vi "Simple Server.vi"() -> ()   [LabVIEW 2020]
uses:
  source/PV Data/NT Scalar (Numeric)/NT Scalar (Numeric).lvclass
  C:/Users/eyw68381/source/repos/pvaccess-labview/labview/source/PV Data/NT Scalar/NT Scalar.lvclass
  C:/Users/eyw68381/source/repos/pvaccess-labview/labview/source/PV Data/NT Base/NT Base.lvclass
  source/PV Data/NT Scalar/NT Scalar.lvclass
  source/PV Data/PV Data/PV Data.lvclass
  source/Server/Server/Server.lvclass
  source/Server/Source/Source.lvclass
  7054ff5f-c778-4b9f-bf9e-4a55a1cdcc59.vi
  4fabb87d-4e15-4188-883f-208453235fd8.vi
  6c06fff3-e822-4e92-b24f-bdc271668697.vi
  0073a8bc-0586-4490-b945-e374f2b6411c.vi
  50f37ae9-e558-497d-927d-4042e789ec73.vi
panel:
  in  "PV name":string="DEV:SIMPLE_TEST"
  out "timestamp":timestamp
  in  "Value":dbl min=0.0 max=10.0 step=0.5 format="%.3f"
  in  "Increment":bool
  in  "stop":bool
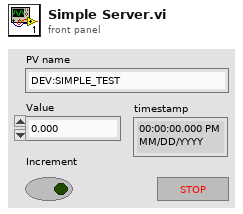
[diagram p1: front panel]
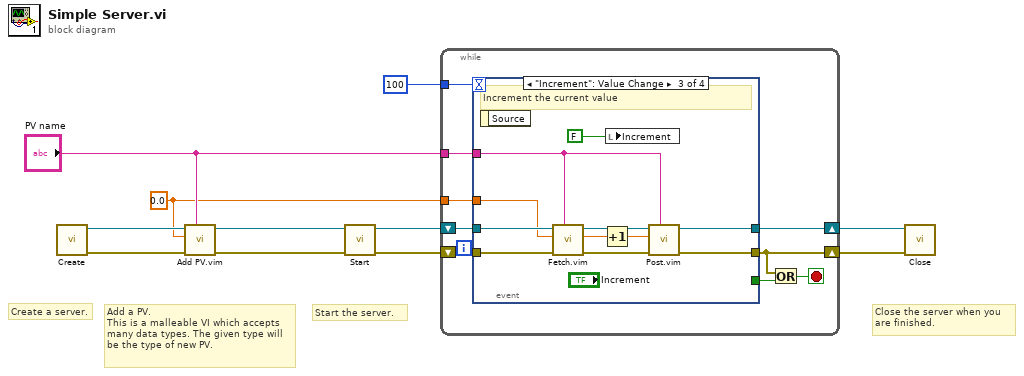
[diagram p0: block diagram]
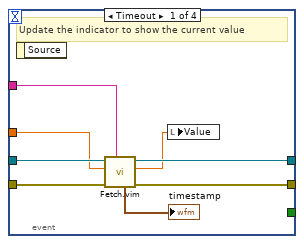
[diagram p2: hidden frame]
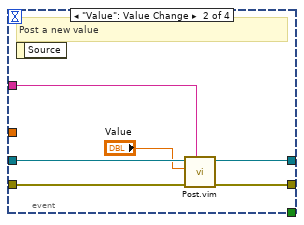
[diagram p3: hidden frame]
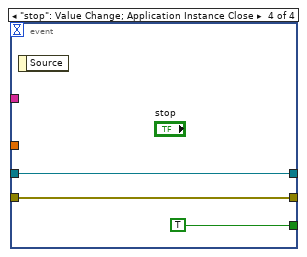
[diagram p4: hidden frame]
diagram:
  w1 = 0.0
  # "Close the server when you are finished."
  # "Start the server."
  # "Add a PV.\nThis is a malleable VI which accepts many data types. The given type will be the type of new PV."
  # "Create a server."
  n1 = call "Create.vi"() -> ("error out"=w2:errorcluster, "Server out"=w8:refnum<class "Server.lvclass">)  [unwired: 10 in]
  n2 = call "Add PV.vim"("PV name"="PV name", "error in"=w2, "initial value"=w1, "Server in"=w8) -> ("error out"=w6:errorcluster, "Server out"=w5:refnum<class "Server.lvclass">)  [unwired: 4 in, 2 out]
  n3 = call-dynamic "Start.vi"("error in (no error)"=w6, "Server in"=w5) -> ("error out"=w3:errorcluster, "Server out"=w4:refnum<class "Server.lvclass">)  [unwired: 8 in]
  n4 = while {
    tunnel: "PV name" -> [w19]
    shift-right: [w17] -> w9
    shift-left: w4 -> [w18]
    shift-right: [w14] -> w10
    shift-left: w3 -> [w20]
    tunnel: 100 ("Numeric") -> [w13]
    tunnel: w1 -> [w12]
    stop <- w15 stop-if-true
    n5 = event shown="[2] \"Increment\": Value Change" {
      selector: _ -> [_ _ _ _]
      dyn-events: _ -> [_ _ _ _]
      timeout: w13 -> [_ _ _ _]
      tunnel: w20 -> [w28 w34 w45 w47]
      tunnel: w19 -> [w23 w33 w38 _]
      tunnel: w18 -> [w27 w32 w44 w46]
      tunnel: [w25 w30 w36 w47] -> w14
      tunnel: [w26 w31 w37 w46] -> w17
      tunnel: [_ _ _ TRUE] -> w16
      tunnel: w12 -> [w21 _ w35 _]
      event Timeout {
        # "Update the indicator to show the current value"
        n6 = event-data() -> ()  [unwired: 1 in, 1 out]
        n7 = call "Fetch.vim"("PV name"=w23, "error in"=w28, "default"=w21, "Server in"=w27) -> ("error out"=w25:errorcluster, "value"=w24:dbl, "Server out"=w26:refnum<class "Server.lvclass">, "timestamp"=→"timestamp":timestamp)  [unwired: 4 in]
        n8 = local write "Value"(w24) -> ()
      }
      event "Value": Value Change {
        # "Post a new value"
        n9 = event-data() -> ()  [unwired: 1 in, 1 out]
        n10 = call "Post.vim"("PV name"=w33, "error in"=w34, "value in"="Value", "Server in"=w32) -> ("error out"=w30:errorcluster, "Server out"=w31:refnum<class "Server.lvclass">)  [unwired: 5 in, 1 out]
      }
      event "Increment": Value Change {
        # "Increment the current value"
        n11 = event-data() -> ()  [unwired: 1 in, 1 out]
        n12 = call "Fetch.vim"("PV name"=w38, "error in"=w45, "default"=w35, "Server in"=w44) -> ("error out"=w41:errorcluster, "value"=w42:dbl, "Server out"=w39:refnum<class "Server.lvclass">)  [unwired: 4 in, 1 out]
        n13 = Increment(x=w42) -> (x+1=w40:dbl)
        n14 = local write "Increment"(FALSE ("Increment")) -> ()
        n15 = call "Post.vim"("PV name"=w38, "error in"=w41, "value in"=w40, "Server in"=w39) -> ("error out"=w36:errorcluster, "Server out"=w37:refnum<class "Server.lvclass">)  [unwired: 5 in, 1 out]
      }
      event "stop": Value Change; Application Instance Close {
        n16 = event-data() -> ()  [unwired: 1 in, 1 out]
      }
    }
    n17 = Or(x=w14, y=w16) -> (x .or. y?=w15:bool)
  }
  n18 = call-dynamic "Close.vi"("error in"=w10, "Server in"=w9) -> ()  [unwired: 9 in, 1 out]
